vi "Layer Scan V6.vi"() -> ()   [LabVIEW 2025]
uses:
  <vilib>/DAQmx/create/channels.llb/DAQmx Create Channel (AO-Voltage-Basic).vi
  <vilib>/DAQmx/miscellaneous.llb/DAQmx Fill In Error Info.vi
  <vilib>/DAQmx/write.llb/DAQmx Write (Analog 1D DBL NChan 1Samp).vi
  <instrlib>/niScope/Configure/Trigger/niScope Configure Trigger Edge.vi
  <instrlib>/niScope/Configure/Trigger/niScope Configure Trigger Immediate.vi
  <instrlib>/niScope/Acquire/Fetch/niScope Multi Fetch.vi
panel:
  in  "Digitizer Channel":string
  in  "Min Record Length":i32=1000
  out "Waveform Graph 2":dbl[](graph) caption="averaged wfm"
  in  "Enforce Realtime":bool=TRUE
  out "Waveform Graph":dbl[][](graph)
  in  "Min. Sample Rate":dbl=1000000.0 format="%#_6p"
  in  "Trigger Type":u16(ring) items=["Edge", "Immediate"]
  in  "Timeout (s)":dbl=5.0 caption="Timeout(s)" format="%.2f"
  in  "Coupling":u16(ring)=1 caption="Trigger Coupling" items=["AC"=0, "DC"=1, "HF Reject"=3, "LF Reject"=4, "AC Plus HF Reject"=1001]
  in  "Trigger Source":string(combo)="0"
  in  "Stop Button":bool
  in  "Vertical Coupling":i32(ring)=1 items=["AC", "DC", "Ground"]
  in  "Num. averages":i32=64
  in  "Resource Name":refnum<k15>="Dev1" caption="Resource Name(s)"
  in  "Simulate?":bool
  out "decimated array 2":dbl[](array[numeric])
  out "decimated array":dbl[](array[numeric])
  out "Y coord filename":i32
  out "x coord file name":i32
  out "Filename Out":path
  in  "Data File Name":path
  in  "Data folder Path":path
  in  "X offset":dbl
  in  "Y offset":dbl
  in  "step":dbl
  in  "Y Count":dbl
  in  "X Count":dbl
  # "Channels and Destinations"
  # "CONFIGURE SCAN"
  # "Constant Parameters"
  # "offset -> dimensions\n10 mm ~= 70 units\n1.5 mm ~= 10 units"
  # "Wave Propagation and Signal Strength Scan Guide"
  # "Signal Strength Scan Only Guide"
  # "1. 'Digitizer Channel' - type in '0,1'\n\n2. 'Resource name' same as SS scan\n\n3. Define data file destination and name\n\n4. Ensure 'Trigger type is set to 'Edge' \n\n5. Choose sample rate. (MAX 2.5 Gs/s)\n\n6. X and Y count must be non-zero\n\n7. Set scan starting offset (from center)\n\n8. Select step size\n\n9. Set 'Num. Averages' to desired value (based on noise).\nWill increase time to finish scan"
  # "1. 'Digitizer Channel' - type in '1'\n\n2. 'Resource Name' - select PXI1Slot2 (visible in NI MAX)\n\n3. Copy and Paste the full path to your data folder\n\n4. Choose a name for your data files\n\n5. Ensure 'Trigger Type' is set to 'Immediate'\n\n6. Choose a sample rate (arbitrary for signal strength)\n\n7. Ensure your count for X and Y axes are NON-ZERO\n\n8. Set the scan starting point by using the 'offset' controls\n\n9. Pick your 'distance' between each point (if your offset coordinate\nstarts at the MAXIMUM coordinates, your 'step' shoud be negative).\ne.g. offset  = (700, 500), then step will have to be (-10).\n\n10. For 'Num. Averages', set to 1. (no need to average because noise isnt a factor)."
  # "General Tips"
  # "1. To have an idea of where youre scanning, play with the offsets using X and Y count == 1\nUsing the SS scan guide\n\n2. Your scan area along each axis will be equal to (X/Y count * Step). \nThe unit is Volts/100 signalled to the ."
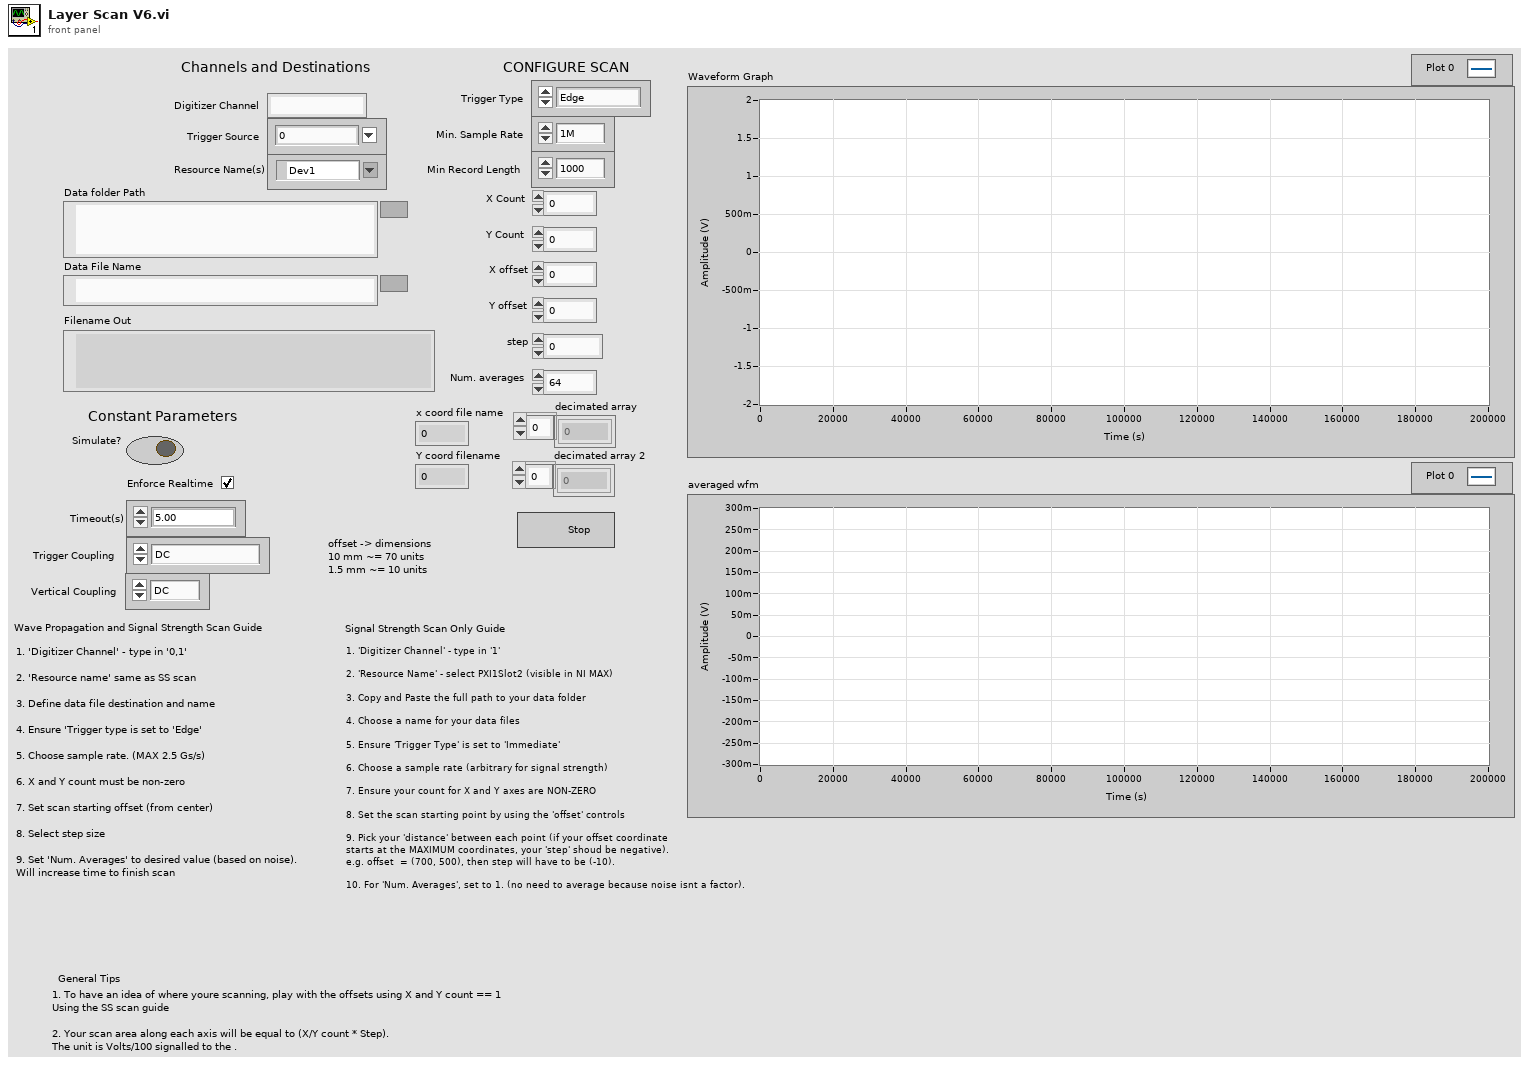
[diagram p1: front panel]
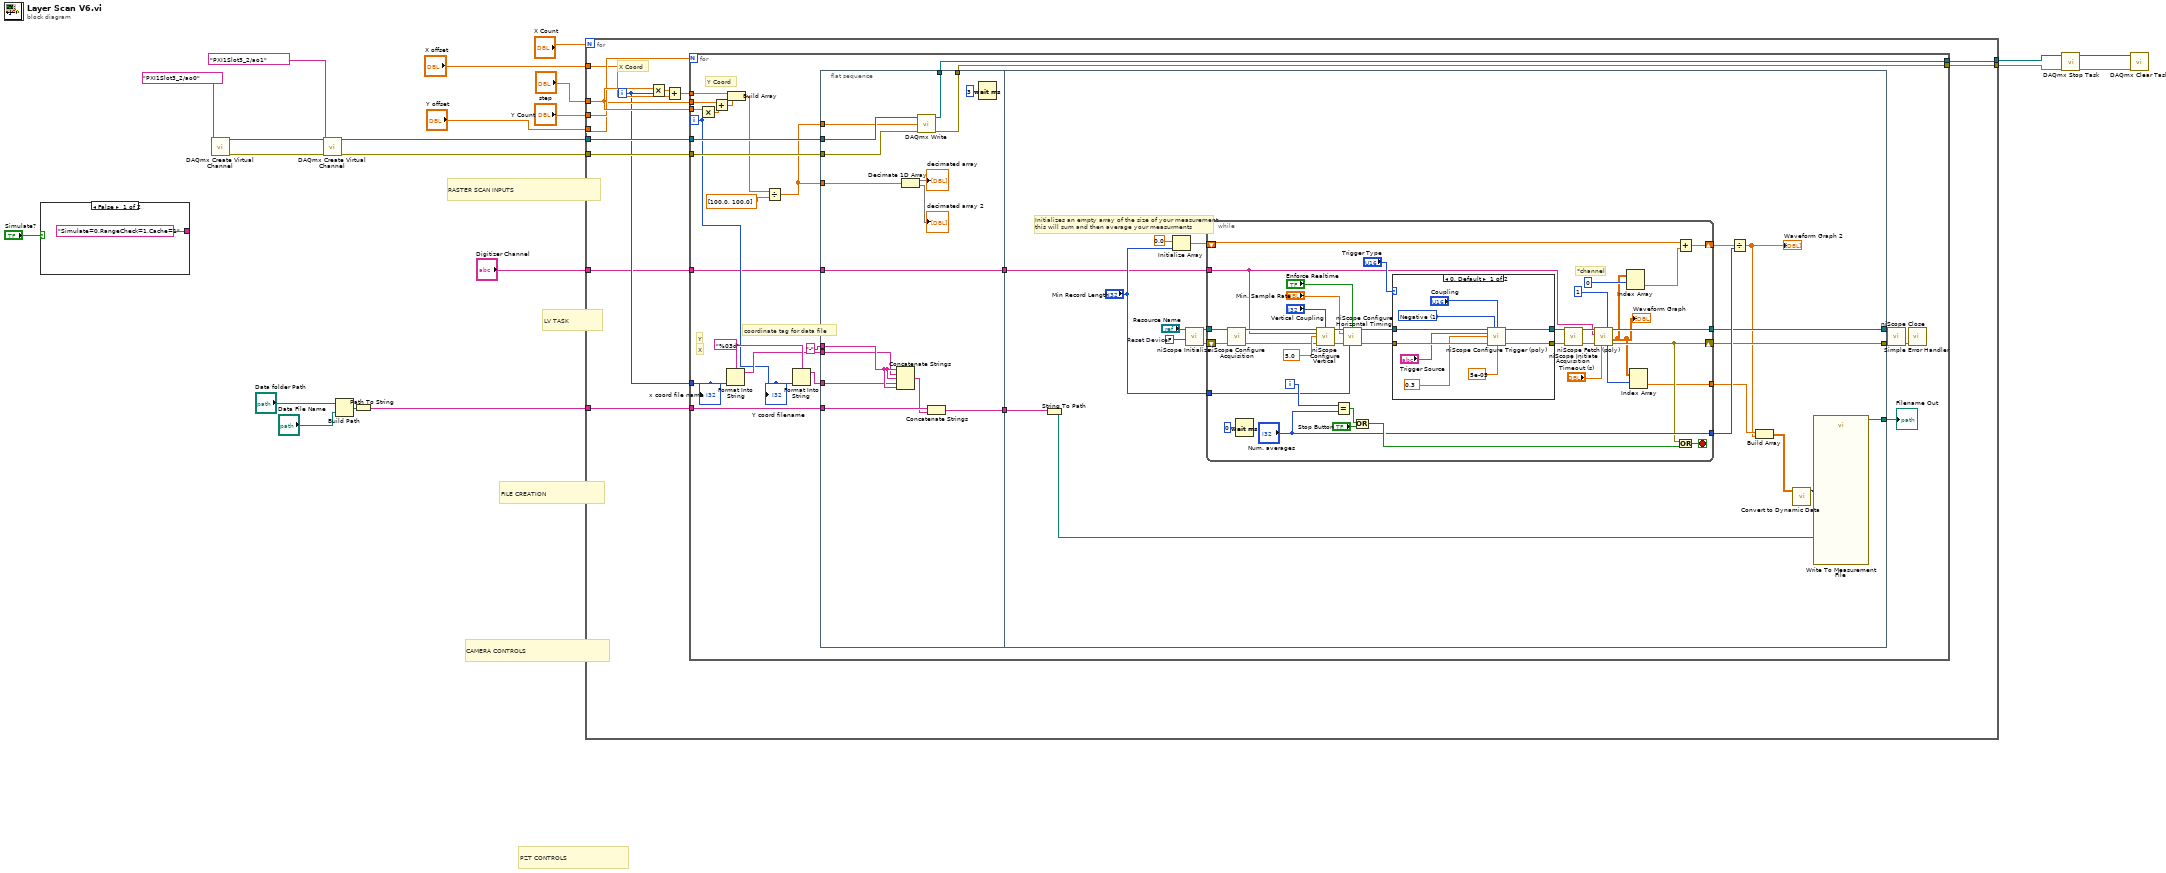
[diagram p0: block diagram]
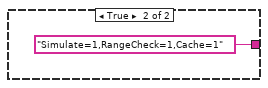
[diagram p2: hidden frame]
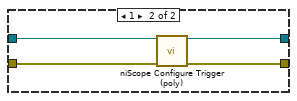
[diagram p3: hidden frame]
diagram:
  # "FILE CREATION"
  # "PZT CONTROLS"
  # "CAMERA CONTROLS"
  # "LV TASK"
  # "RASTER SCAN INPUTS"
  n1 = case shown="False" "Simulate?" {
    tunnel: ["Simulate=0,RangeCheck=1,Cache=1" ("option string") "Simulate=1,RangeCheck=1,Cache=1" ("option string")] -> _
    frame False {
    }
    frame True {
    }
  }
  n2 = call-poly <vilib>:"DAQmx Create Virtual Channel.vi"("physical channels"=tag "PXI1Slot3_2/ao0") -> ("task out"=w14:refnum<k21>, "error out"=w13:errorcluster)  [unwired: 13 in]
  n3 = call-poly <vilib>:"DAQmx Create Virtual Channel.vi"("task in"=w14, "physical channels"=tag "PXI1Slot3_2/ao1", "error in"=w13) -> ("task out"=w12:refnum<k21>, "error out"=w11:errorcluster)  [unwired: 11 in]
  n4 = Build Path(base path="Data folder Path", name or relative path="Data File Name") -> (appended path=w4:path)
  n5 = Path To String(path=w4) -> (string=w3:string)
  n6 = for {
    N: "X Count" -> [_]
    tunnel: "step" -> [w36]
    tunnel: "Y Count" -> [w35]
    tunnel: "Y offset" -> [w34]
    tunnel: "X offset" -> [w32]
    tunnel: w12 -> [w30]
    tunnel: w11 -> [w29]
    tunnel: [w28] -> w10
    tunnel: [w27] -> w9
    tunnel: w3 -> [w26]
    tunnel: "Digitizer Channel" -> [w24]
    i -> [w25]
    # "X Coord"
    n7 = Multiply(x=w36, y=w25) -> (x*y=w33:dbl)
    n8 = Add(x=w33, y=w32) -> (x+y=w31:dbl)
    n9 = for {
      N: w35 -> [_]
      tunnel: w36 -> [w62]
      tunnel: w34 -> [w60]
      tunnel: w31 -> [w59]
      tunnel: w30 -> [w57]
      tunnel: w29 -> [w56]
      tunnel: [w54] -> w28
      tunnel: [w53] -> w27
      tunnel: w26 -> [w48]
      tunnel: w25 -> [w45]
      tunnel: w24 -> [w41]
      i -> [w44]
      w52 = "%03d" ("format string")
      # "coordinate tag for data file"
      # "X"
      # "Y"
      # "Y Coord"
      n10 = Multiply(x=w62, y=w44) -> (x*y=w61:dbl)
      n11 = Add(x=w60, y=w61) -> (x+y=w58:dbl)
      n12 = Format Into String(format string=w52, w45) -> (resulting string=w50:string)  [unwired: 2 in, 1 out]
      n13 = Build Array(w59, w58) -> (w55:dbl[])
      n14 = Divide(x=w55, y=dbl[] [100.0, 100.0]) -> (x/y=w43:dbl[])
      n15 = Format Into String(format string=w52, w44) -> (resulting string=w49:string)  [unwired: 2 in, 1 out]
      n16 = flat-sequence {
        tunnel: w57 -> [w77]
        tunnel: w56 -> [w76]
        tunnel: [w75] -> w54
        tunnel: [w74] -> w53
        tunnel: "-" ("string") -> [w73]
        tunnel: w50 -> [w72]
        tunnel: w49 -> [w71]
        tunnel: w48 -> [w70]
        tunnel: [w68] -> w47
        tunnel: w43 -> [w67]
        tunnel: w43 -> [w66]
        tunnel: w41 -> [w63]
        tunnel: [w63] -> w40
        tunnel: [w97] -> w42
        tunnel: [w84] -> w38
        tunnel: [w83] -> w37
        tunnel: w40 -> [w85]
        tunnel: w47 -> [w96]
        frame #0 {
          n17 = Concatenate Strings(w73, w72, w73, w71, w73) -> (w69:string)
          n18 = Decimate 1D Array(w66) -> (→"decimated array":dbl[], →"decimated array 2":dbl[])
          n19 = call-poly <vilib>:"DAQmx Write.vi"("task/channels in"=w77, "data"=w67, "error in"=w76) -> ("task out"=w75:refnum<k21>, "error out"=w74:errorcluster)  [unwired: 10 in, 1 out]
          n20 = Concatenate Strings(w70, w69) -> (w68:string)
          n21 = Wait (ms)(milliseconds to wait=u32 3) -> ()  [unwired: 1 out]
        }
        frame #1 {
          w94 = FALSE  # Reset Device
          # "Initializes an empty array of the size of your measurement,\nthis will sum and then average your measurments"
          n22 = String To Path(string=w96) -> (path=w95:path)
          n23 = Initialize Array(0.0 ("element"), "Min Record Length") -> (w88:dbl[])
          n24 = call <instrlib>:"niScope Initialize.vi"("resource name"="Resource Name", "reset device"=w94) -> ("instrument handle"=w92:refnum<k15>, "error out"=w91:errorcluster)  [unwired: 12 in]
          n25 = while {
            tunnel: w92 -> [w121]
            tunnel: [w105] -> w84
            shift-right: [w104] -> w83
            shift-left: w91 -> [w120]
            tunnel: ["Num. averages"] -> w90
            shift-right: [w113] -> w89
            shift-left: w88 -> [w112]
            tunnel: "Min Record Length" -> [w111]
            tunnel: w85 -> [w106]
            tunnel: [w98] -> w82
            i -> [w115]
            stop <- w122 stop-if-true
            # "*channel"
            n26 = call <instrlib>:"niScope Configure Acquisition.vi"("instrument handle"=w121, "error in"=w120) -> ("instrument handle out"=w127:refnum<k15>, "error out"=w128:errorcluster)  [unwired: 12 in]
            n27 = Wait (ms)(milliseconds to wait=u32 0 ("millisecond multiple")) -> ()  [unwired: 1 out]
            n28 = call <instrlib>:"niScope Configure Vertical.vi"("instrument handle"=w127, "vertical coupling"="Vertical Coupling", "channels"=w106, "vertical range"=5.0 ("Vertical Range (V)"), "error in"=w128) -> ("instrument handle out"=w132:refnum<k15>, "error out"=w133:errorcluster)  [unwired: 9 in]
            n29 = Equal?(x=w115, y="Num. averages") -> (x = y?=w118:bool)
            n30 = call <instrlib>:"niScope Configure Horizontal Timing.vi"("instrument handle"=w132, "enforce realtime"="Enforce Realtime", "min sample rate"="Min. Sample Rate", "error in"=w133, "min record length"=w111) -> ("instrument handle out"=w126:refnum<k15>, "error out"=w125:errorcluster)  [unwired: 9 in]
            n31 = Or(x=w118, y="Stop Button") -> (x .or. y?=w116:bool)
            n32 = case shown="0, Default" "Trigger Type" {
              tunnel: w126 -> [w142 w146]
              tunnel: w125 -> [w141 w143]
              tunnel: [w140 w145] -> w108
              tunnel: [w139 w144] -> w107
              frame 0, Default {
                w137 = u16 1 items=["Positive", "Negative"] ("Trigger Slope")
                n33 = call-poly <instrlib>:"niScope Configure Trigger (poly).vi"("instrument handle"=w142, "trigger slope"=w137, "trigger coupling"="Coupling", "trigger source"="Trigger Source", "trigger level"=0.3 ("Trigger Level"), "error in"=w141, "trigger delay"=5e-05) -> ("instrument handle out"=w140:refnum<k15>, "error out"=w139:errorcluster)  [unwired: 7 in]
              }
              frame 1 {
                n34 = call-poly <instrlib>:"niScope Configure Trigger (poly).vi"("instrument handle"=w146, "error in"=w143) -> ("instrument handle out"=w145:refnum<k15>, "error out"=w144:errorcluster)  [unwired: 12 in]
              }
            }
            n35 = call <instrlib>:"niScope Initiate Acquisition.vi"("instrument handle"=w108, "error in"=w107) -> ("instrument handle out"=w109:refnum<k15>, "error out"=w110:errorcluster)  [unwired: 12 in]
            n36 = call-poly <instrlib>:"niScope Fetch (poly).vi"("timeout"="Timeout (s)", "error in"=w110, "channels"=w106, "instrument handle"=w109) -> ("error out"=w104:errorcluster, "wfm"=w100:dbl[][], "instrument handle out"=w105:refnum<k15>)  [unwired: 4 in, 1 out]
            "Waveform Graph" <- w100
            n37 = Index Array(array=w100, index (row)=0) -> (element=w102:dbl[])  [unwired: 1 in]
            n38 = Index Array(array=w100, index (row)=1) -> (element=w98:dbl[])  [unwired: 1 in]
            n39 = Add(x=w112, y=w102) -> (x+y=w113:dbl[])
            n40 = Or(x=w104, y=w116) -> (x .or. y?=w122:bool)
          }
          n41 = Divide(x=w89, y=w90) -> (x/y=w81:dbl[])
          "Waveform Graph 2" <- w81
          n42 = Build Array(w82, w81) -> (w80:dbl[][])
          n43 = call "Convert to Dynamic Data"("2D Array"=w80) -> ("Dynamic Data Type"=w79:dynamicdata)  [unwired: 3 in]
          n44 = call "Write To Measurement File"("Signals"=w79, "Filename"=w95) -> ("Filename Out"=w97:path)  [unwired: 15 in, 2 out]
        }
      }
      n45 = call <instrlib>:"niScope Close.vi"("instrument handle"=w38, "error in"=w37) -> ("error out"=w39:errorcluster)  [unwired: 13 in]
      n46 = call <vilib>:"Simple Error Handler.vi"("error in (no error)"=w39) -> ()  [unwired: 4 in, 5 out]
      "Filename Out" <- w42
      "x coord file name" <- w45
      "Y coord filename" <- w44
    }
  }
  n47 = call <vilib>:"DAQmx Stop Task.vi"("task/channels in"=w10, "error in"=w9) -> ("task out"=w8:refnum<k21>, "error out"=w7:errorcluster)  [unwired: 12 in]
  n48 = call <vilib>:"DAQmx Clear Task.vi"("task in"=w8, "error in"=w7) -> ()  [unwired: 13 in, 1 out]
